vi "Filter Area ROIContours.vi"(8 "error in (no error)":errorcluster, 11 "Analyze BaseClass in":refnum<class "Analyze BaseClass.lvclass">) -> (0 "error out":errorcluster, 2 "ROI of Area type":T1 {"Contours"."Type" items=["No Selection", "Point", "Line", "Rectangle", "Oval", "Polygon", "Freehand Region", "Annulus", "Unused2", "Unused3", "Broken Line", "Freehand Line", "Rotated Rectangle"]}, 3 "Analyze BaseClass out":refnum<class "Analyze BaseClass.lvclass">)   [LabVIEW 2009, in "Analyze BaseClass.lvclass"]
uses:
  Analyze BaseClass.lvclass
  Analyze BaseClass.lvclass/Analyze BaseClass.ctl
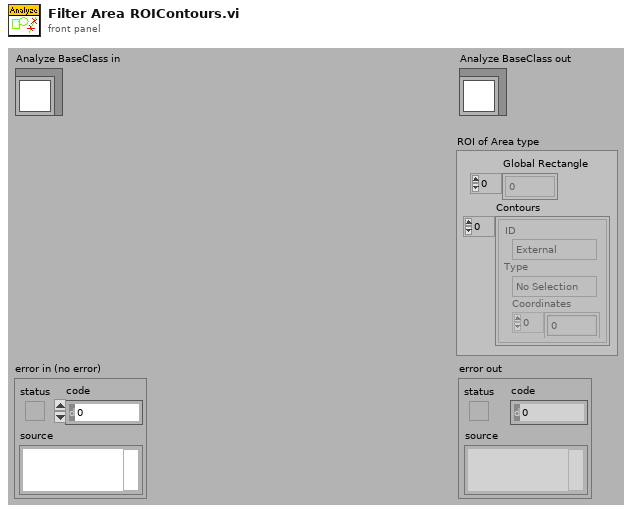
[diagram p1: front panel]
types:
  T1 = typedef "ROI Descriptor" = cluster{"Global Rectangle":i32[], "Contours":cluster{"ID":enum32{"External", "Internal"}, "Type":u32, "Coordinates":i32[]}[]}
  T2 = cluster{"ID":enum32{"External", "Internal"}, "Type":u32, "Coordinates":i32[]}[]
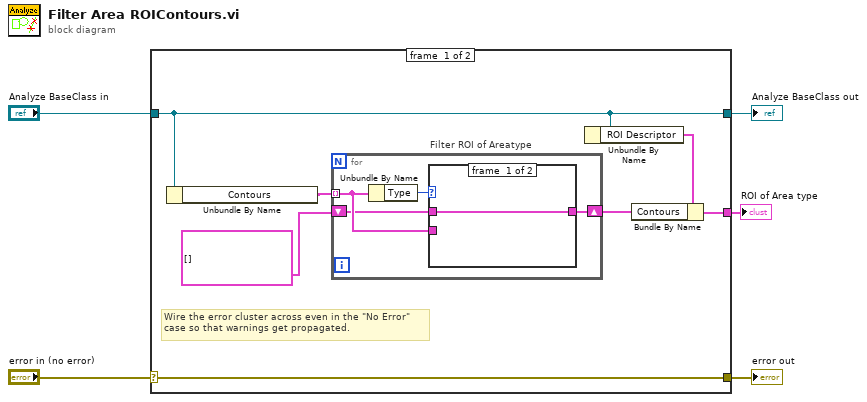
[diagram p0: block diagram]
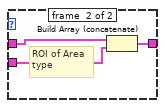
[diagram p2: hidden frame]
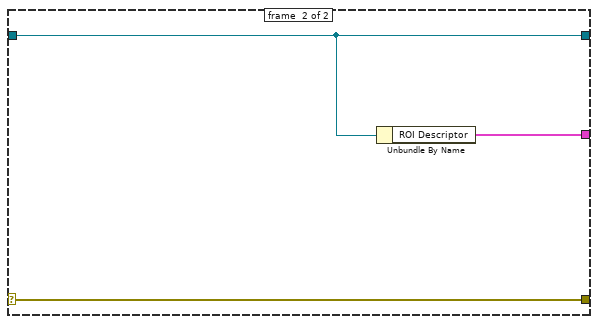
[diagram p3: hidden frame]
diagram:
  n1 = case shown="No Error" "error in (no error)" {
    selector: "error in (no error)" -> [w12 w23]
    tunnel: [w12 w23] -> w4
    tunnel: [w7 w22] -> w2
    tunnel: "Analyze BaseClass in" -> [w7 w22]
    tunnel: [w8 w21] -> w1
    frame #0 {
      # "Wire the error cluster across even in the \"No Error\"\ncase so that warnings get propagated."
      n2 = Unbundle By Name(w7) -> ("Contours"=w9:T2)
      n3 = for "Filter ROI of Areatype" {
        tunnel: w9 -> [w15] mode=indexing
        shift-right: [w14] -> w10
        shift-left: T2 [] -> [w13]
        n4 = Unbundle By Name(w15) -> ("Type"=w16:u32)
        n5 = case shown="3..7, 12" w16 {
          tunnel: w15 -> [_ w20]
          tunnel: [w17 w19] -> w14
          tunnel: w13 -> [w17 w18]
          frame #0 {
          }
          frame #1 {
            # "ROI of Area\ntype"
            n6 = Build Array (concatenate)(w18, w20) -> (w19:T2)
          }
        }
      }
      n7 = Unbundle By Name(w7) -> ("ROI Descriptor"=w6:T1)
      n8 = Bundle By Name(cluster=w6, "Contours"=w10) -> (w8:T1)
    }
    frame #1 {
      n9 = Unbundle By Name(w22) -> ("ROI Descriptor"=w21:T1)
    }
  }
  "error out" <- w4
  "Analyze BaseClass out" <- w2
  "ROI of Area type" <- w1
